vi "Read Calculated limit Config.vi"(8 "error in (no error)":errorcluster) -> (0 "error out":errorcluster, 3 "Cal Limits":T1[](array[typedef]))   [LabVIEW 2018]
uses:
  Controls/Calculated Limits.ctl
  <vilib>/Utility/xml.llb/Read From XML File(string).vi
panel:
  # "Lower Fault"
  # "Event"
  # "Lower Warning"
  # "Higher Warning"
  # "Higher Fault"
  # "Event"
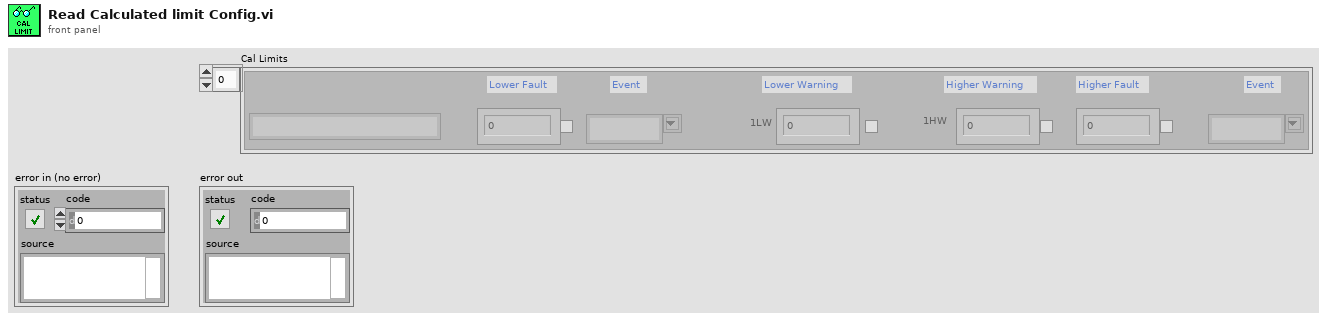
[diagram p1: front panel]
types:
  T1 = typedef "Calculated Limits.ctl" = cluster{"1LF":dbl, "1HW select":bool, "1LW select":bool, "1LF select":bool, "1HW":dbl, "1LW":dbl, "1HF":dbl, "1HF select":bool, "CH1":string, "1_LF_EVENT":string, "1_HF_EVENT":string}
  T2 = typedef "Limit Paths.ctl" = cluster{"Limit 1 Config Path":path, "Limit 2 Config Path ":path, "Limit 3 Config Path ":path, "Limit 4 Config Path ":path, "Limit 5 Config Path ":path, "Limit 6 Config Path ":path, "CallimitPath ":path}
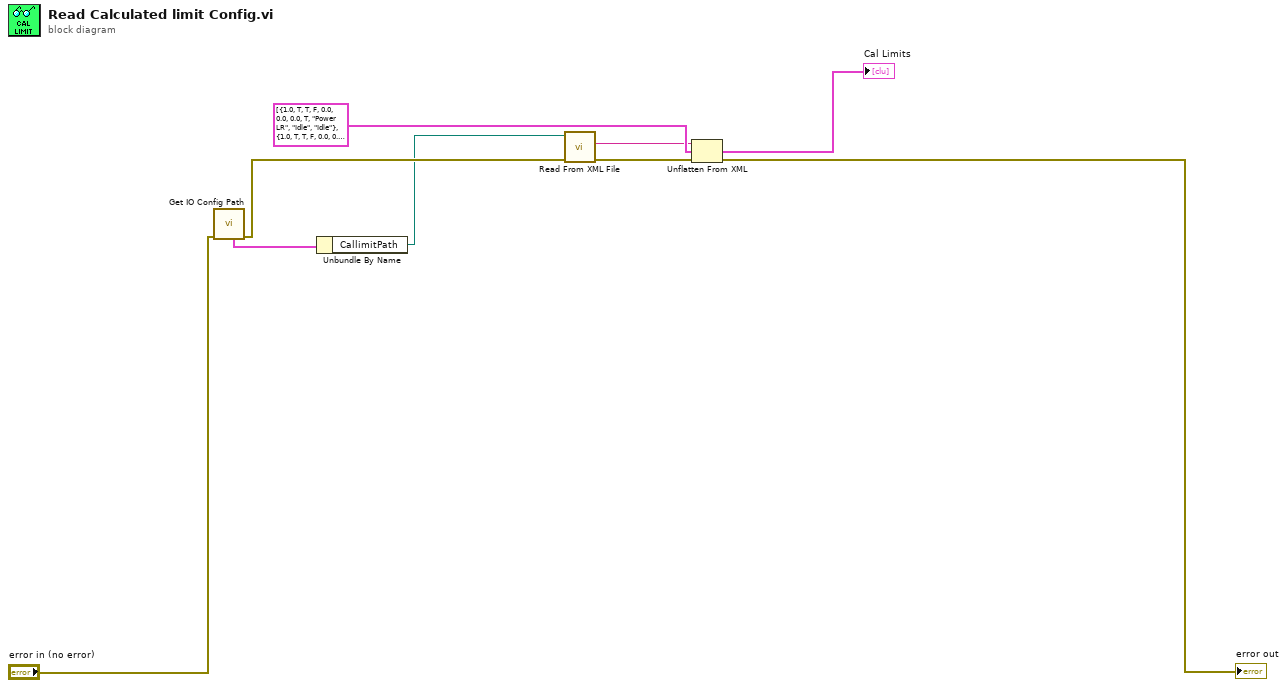
[diagram p0: block diagram]
diagram:
  n1 = call "Get IO Config Path.vi"("error in (no error)"="error in (no error)") -> ("error out"=w7:errorcluster, "Limit Path"=w5:T2)  [unwired: 5 in, 4 out]
  n2 = Unbundle By Name(w5) -> ("CallimitPath"=w6:path)
  n3 = call-poly <vilib>:"Read From XML File.vi"("error in (no error)"=w7, "XML File Path"=w6) -> ("error out"=w1:errorcluster, "XML Elements"=w2:string)  [unwired: 7 in, 1 out]
  n4 = Unflatten From XML(xml string=w2, type=T1[] [{"1LF"=1.0, "1HW select"=TRUE, "1LW select"=TRUE, "1LF select"=FALSE, "1HW"=0.0, "1LW"=0.0, "1HF"=0.0, "1HF select"=TRUE, "CH1"="Power LR", "1_LF_EVENT"="Idle", "1_HF_EVENT"="Idle"}, {"1LF"=1.0, "1HW select"=TRUE, "1LW select"=TRUE, "1LF select"=FALSE, "1HW"=0.0, "1LW"=0.0, "1HF"=0.0, "1HF select"=TRUE, "CH1"="Power H", "1_LF_EVENT"="Idle", "1_HF_EVENT"="Idle"}] ("Cal Limits"), error in (no error)=w1) -> (value=→"Cal Limits":T1[], error out=→"error out":errorcluster)
